vi "Write Place point.vi"(8 "error in (no error)":errorcluster, 9 "Text Point":cluster{"x":i32, "y":i32}, 10 "Icon Point":cluster{"x":i32, "y":i32}, 11 "Control in":refnum<class "Control.lvclass">) -> (0 "error out":errorcluster, 3 "Control out":refnum<class "Control.lvclass">)   [LabVIEW 2013, in "uitools_Control.lvlib" / "Control.lvclass"]
uses:
  Control.lvclass
  Control.lvclass/Control.ctl
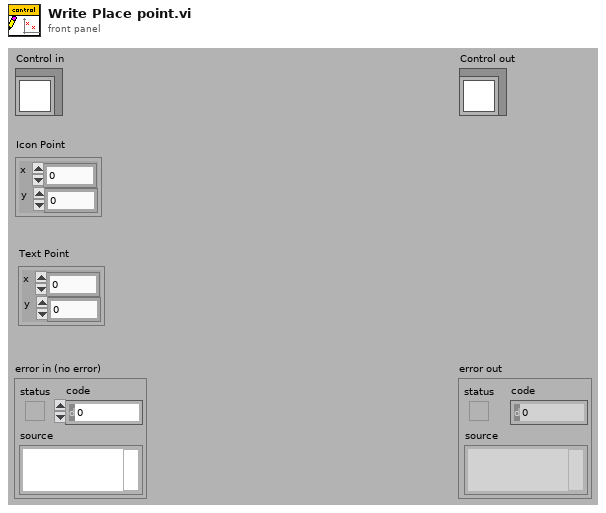
[diagram p1: front panel]
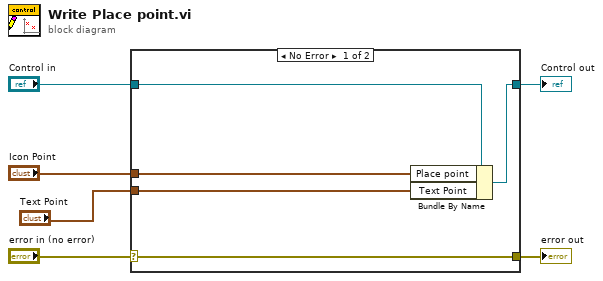
[diagram p0: block diagram]
diagram:
  n1 = case shown="No Error" "error in (no error)" {
    selector: "error in (no error)" -> [w11 w12]
    tunnel: [w11 w12] -> w5
    tunnel: [w9 w13] -> w3
    tunnel: "Control in" -> [w10 w13]
    tunnel: "Icon Point" -> [w8 _]
    tunnel: "Text Point" -> [w7 _]
    frame No Error {
      n2 = Bundle By Name(cluster=w10, "Place point"=w8, "Text Point"=w7) -> (w9:refnum<class "Control.lvclass">)
    }
    frame Error {
    }
  }
  "error out" <- w5
  "Control out" <- w3
